vi "BooleanNotifier Get.vi"(8 "error in (no error)":errorcluster, 11 "BooleanNotifier in":refnum<class "BooleanNotifier.lvclass">) -> (0 "error out":errorcluster, 2 "Last boolean out":bool, 3 "BooleanNotifier out":refnum<class "BooleanNotifier.lvclass">)   [LabVIEW 2018, in "BooleanNotifier.lvclass"]
uses:
  BooleanNotifier.lvclass
  BooleanNotifier.lvclass/BooleanNotifier.ctl
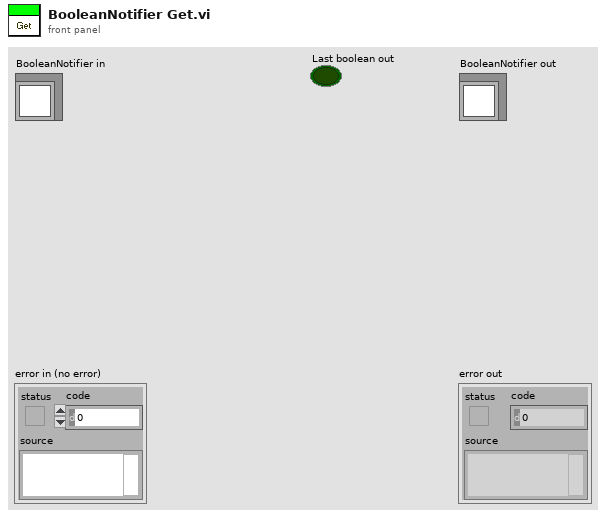
[diagram p1: front panel]
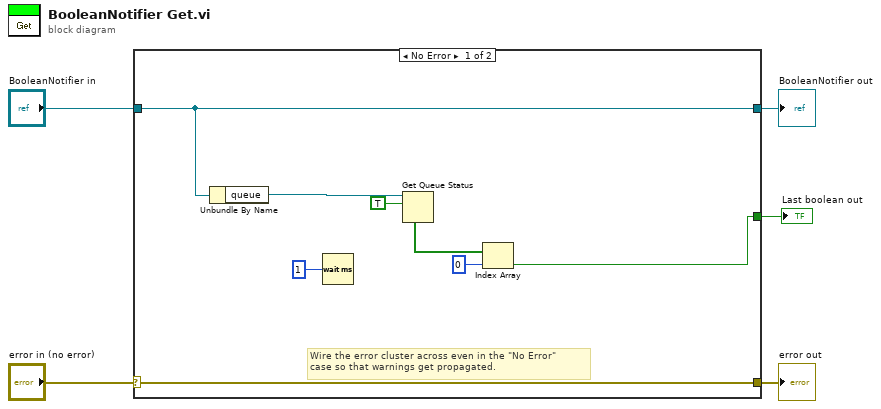
[diagram p0: block diagram]
diagram:
  n1 = case shown="No Error" "error in (no error)" {
    selector: "error in (no error)" -> [w13 w15]
    tunnel: [w13 w15] -> w4
    tunnel: [w12 w14] -> w2
    tunnel: "BooleanNotifier in" -> [w12 w14]
    tunnel: [w8 _] -> w1
    frame No Error {
      # "Wire the error cluster across even in the \"No Error\"\ncase so that warnings get propagated."
      n2 = Unbundle By Name(w12) -> ("queue"=w11:refnum<queue>)
      n3 = Wait (ms)(milliseconds to wait=u32 1) -> ()  [unwired: 1 out]
      n4 = Get Queue Status(queue=w11, return elements? (F)=TRUE) -> (elements=w9:bool[])  [unwired: 1 in, 7 out]
      n5 = Index Array(array=w9, index=0) -> (element=w8:bool)
    }
    frame Error {
    }
  }
  "error out" <- w4
  "BooleanNotifier out" <- w2
  "Last boolean out" <- w1
